vi "OEE_SCREEN_2_recolor_stations_over_cycle_time.vi"(1 "over_cycle_time_actual_field_reference":refnum<vi>, 2 "over_cycle_time_actual":string) -> ()   [LabVIEW 2019]
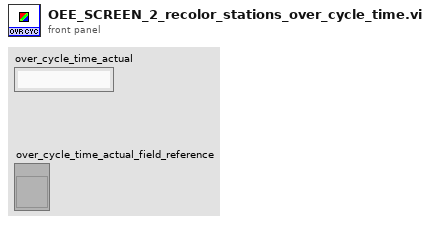
[diagram p1: front panel]
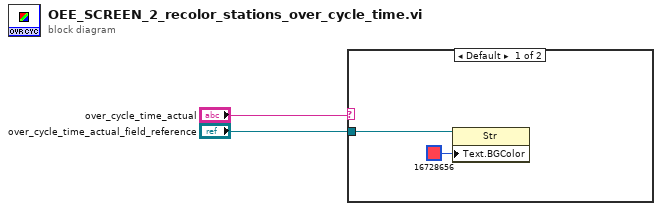
[diagram p0: block diagram]
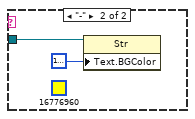
[diagram p2: hidden frame]
diagram:
  n1 = case shown="Default" "over_cycle_time_actual" {
    tunnel: "over_cycle_time_actual_field_reference" -> [w4 w6]
    frame Default {
      n2 = property class="Str"(reference=w4, "Text.BGColor"=u32 16728656) -> ()  [unwired: 1 in, 2 out]
    }
    frame "-" {
      (unwired) u32 16776960
      n3 = property class="Str"(reference=w6, "Text.BGColor"=u32 16777238) -> ()  [unwired: 1 in, 2 out]
    }
  }
